vi "Write_parameter.vi"(8 "error in (no error)":errorcluster caption="entrée d'erreur (pas d'erreur)", 10 "Parameter":string, 11 "Class Instrument Multimeter en entrée":refnum<class "Class Instrument Schielding_Box.lvclass">) -> (0 "error out":errorcluster caption="sortie d'erreur", 3 "Class Instrument Multimeter en sortie":refnum<class "Class Instrument Schielding_Box.lvclass">)   [LabVIEW 2020, in "Library Instrument & Equipement.lvlib" / "Library Instruments.lvlib" / "Class Instrument Schielding_Box.lvclass"]
uses:
  Class Instrument Schielding_Box.lvclass
  Commun VI/TypeDef/Commande Shielding box/Commande Shielding box.ctl
  Shielding box/Class Shielding box (Default)/Class Shielding_ Box (Default).lvclass
  JSON API/JSON Value/Set from JSON string.vi
  Instrument (Default)/Class Instrument (Default).lvclass
  JSON API/JSON Value/JSON Value.lvclass
  Class Instrument Schielding_Box.lvclass/Class Instrument Schielding_Box.ctl
  JSON API/Variant JSON/Variant JSON.lvlib
  JSON API/Get Polymorphic/JSON GetSet.lvlib
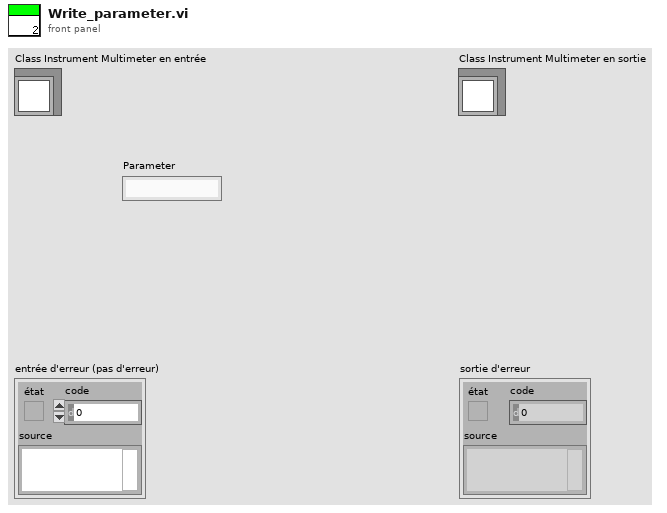
[diagram p1: front panel]
types:
  T1 = typedef "Commande Shielding box.ctl" = cluster{"Device @":string, "Class Shielding_ Box":refnum<class "Class Shielding_ Box (Default).lvclass">}
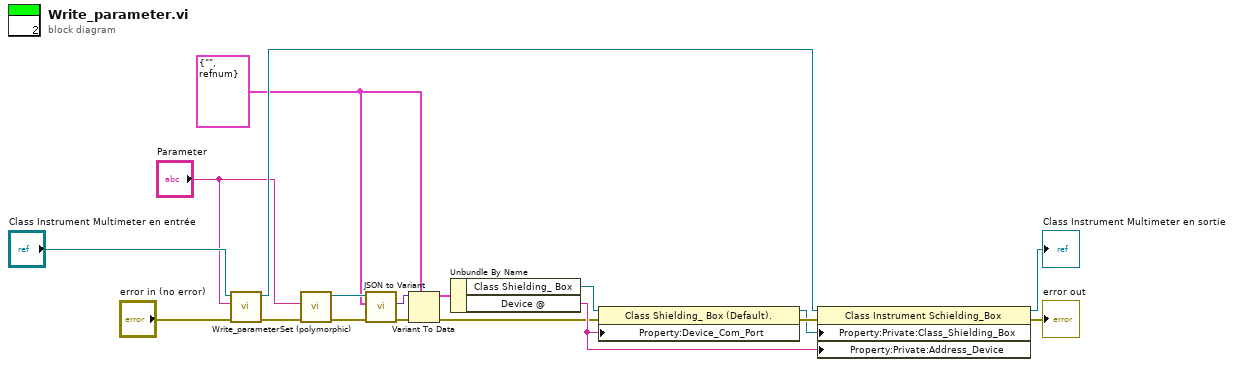
[diagram p0: block diagram]
diagram:
  w3 = T1 {"Device @"="", "Class Shielding_ Box"=refnum} ("Parameter")
  n1 = call-parent "Write_parameter.vi"("error in (no error)"="error in (no error)", "Parameter"="Parameter", "Class Instrument (Default) en entrée"="Class Instrument Multimeter en entrée") -> ("error out"=w10:errorcluster, "Class Instrument (Default) en sortie"=w9:refnum<class "Class Instrument Schielding_Box.lvclass">)  [unwired: 7 in]
  n2 = call-poly "Set (polymorphic).vi"("error in (no error)"=w10, "JSON stream"="Parameter") -> ("error out"=w16:errorcluster, "JSON Value out"=w18:refnum<class "JSON Value.lvclass">)  [unwired: 7 in, 1 out]
  n3 = call "JSON to Variant.vi"("error in (no error)"=w16, "Variant (Data Type)"=w3, "JSON Value"=w18) -> ("error out"=w17:errorcluster, "Variant out"=w15:variant)  [unwired: 7 in]
  n4 = Variant To Data(error in=w17, type=w3, Variant=w15) -> (data=w12:T1, error out=w4:errorcluster)
  n5 = Unbundle By Name(w12) -> ("Class Shielding_ Box"=w1:refnum<class "Class Shielding_ Box (Default).lvclass">, "Device @"=w6:string)
  n6 = property class="Class Shielding_ Box (Default)."(reference=w1, error in=w4, "Property:Device_Com_Port"=w6) -> (reference out=w2:refnum<class "Class Shielding_ Box (Default).lvclass">, error out=w5:errorcluster)
  n7 = property class="Class Instrument Schielding_Box"(reference=w9, error in=w5, "Property:Private:Class_Shielding_Box"=w2, "Property:Private:Address_Device"=w6) -> (reference out=→"Class Instrument Multimeter en sortie":refnum<class "Class Instrument Schielding_Box.lvclass">, error out=→"error out":errorcluster)
